vi "Bundle to Font Settings.vi"(9 "Justification":enum16{"Left", "Center", "Right"}(ring), 11 "Font":T1) -> (3 "Font Settings":T2)   [LabVIEW 2016, in "FontUIP.lvclass"]
uses:
  FontUIP.lvclass
  Font Settings.ctl
  <vilib>/Utility/miscctls.llb/LVFontTypeDef.ctl
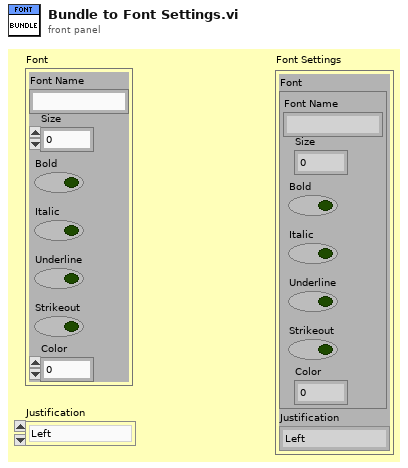
[diagram p1: front panel]
types:
  T1 = typedef "LVFontTypeDef.ctl" = cluster{"Font Name":string, "Size":u16, "Bold":bool, "Italic":bool, "Underline":bool, "Strikeout":bool, "Color":u32}
  T2 = typedef "FontUIP.lvclass/Font Settings.ctl" = cluster{"Font":T1, "Justification":enum16{"Left", "Center", "Right"}}
  T3 = cluster{"Font":T1, "Justification":enum16{"Left", "Center", "Right"}}
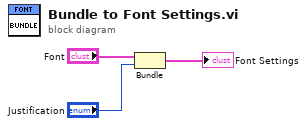
[diagram p0: block diagram]
diagram:
  n1 = Bundle("Font"="Font", "Justification"="Justification") -> (→"Font Settings":T3)  [unwired: 1 in]
